vi "main(Test DQMH modules).vi"() -> ()   [LabVIEW 2018, in "Application.lvlib"] (continued)
        n2137 = Build Array(w5001, w5000, w4999) -> (w5007:T9[])
        n2138 = for {
          tunnel: [w5039] -> w5013 mode=indexing
          shift-right: [w5040] -> w5015
          shift-left: w5008 -> [w5038]
          tunnel: w5007 -> [w5037] mode=indexing
          n2139 = Unbundle By Name(w5037) -> ("command"=w5036:string, "data"=w5035:variant)
          n2140 = call "App enquece.vi"("Priority Enquece"=TRUE, "command data"=w5035, "command"=w5036, "queue in"=w5038) -> ("error out"=w5039:errorcluster, "Queue out"=w5040:refnum<queue>)  [unwired: 6 in]
        }
        n2141 = call "FGV DRV stand.vi"() -> ("Sub-Test.DCV"=w4996:bool)  [unwired: 10 in, 1 out]
        n2142 = case shown="True" w4996 {
          tunnel: [w5026 w5034] -> w5016
          frame False {
            n2143 = Build Array("WaitFor", "MEAS.requestAC") -> (w5026:string[])
          }
          frame True {
            n2144 = Build Array("Test DRV 1", "Test DRV 2", "Test DRV 3", "WaitForC", "MEAS.requestAC") -> (w5034:string[])
          }
        }
        n2145 = Merge Errors(w5013) -> (w5006:errorcluster)
        n2146 = Reverse 1D Array(array=w5016) -> (reversed array=w4995:string[])
        n2147 = for {
          tunnel: w4995 -> [w5046] mode=indexing
          tunnel: [w5045] -> w5012 mode=indexing
          shift-right: [w5044] -> w5014
          shift-left: w5015 -> [w5047]
          tunnel: w5006 -> [w5043]
          n2148 = call "App enquece.vi"("Priority Enquece"=TRUE, "error in (no error)"=w5043, "command"=w5046, "queue in"=w5047) -> ("error out"=w5045:errorcluster, "Queue out"=w5044:refnum<queue>)  [unwired: 6 in]
        }
        n2149 = Merge Errors(w5012) -> (w5011:errorcluster)
        n2150 = Initialize Array(FALSE ("element"), 6 ("dimension size")) -> (w4977:bool[])
        n2151 = Initialize Array(TRUE, 3 ("dimension size")) -> (w4976:bool[])
        n2152 = Replace Array Subset(array=w4977, new element=w4976) -> (w4975:bool[])  [unwired: 1 in]
        n2153 = To Variant(anything=T3."mux10_1_channel1" ("mux10_1(x6)_encode")) -> (Variant=w4992:variant)
        n2154 = To Variant(anything=T4."demux1_10_channel1" ("demux1_10(x6)_encode")) -> (Variant=w4988:variant)
        n2155 = To Variant(anything=w4975) -> (Variant=w4984:variant)
        n2156 = Bundle By Name(cluster=w4981, "command"="MEAS.mux10-1", "data"=w4992) -> (w4987:T9)
        n2157 = Bundle By Name(cluster=w4981, "command"="MEAS.demux1-10", "data"=w4988) -> (w4986:T9)
        n2158 = Bundle By Name(cluster=w4981, "command"="MEAS.eMIC", "data"=w4984) -> (w4983:T9)
        n2159 = Build Array(w4987, w4986, w4983) -> (w5010:T9[])
        n2160 = Reverse 1D Array(array=w5010) -> (reversed array=w5009:T9[])
        n2161 = for {
          tunnel: w5009 -> [w5057] mode=indexing
          tunnel: [w5054] -> w5017 mode=indexing
          tunnel: w5011 -> [w5053]
          tunnel: w5014 -> [w5058]
          n2162 = Unbundle By Name(w5057) -> ("command"=w5056:string, "data"=w5055:variant)
          n2163 = call "App enquece.vi"("Priority Enquece"=TRUE, "error in (no error)"=w5053, "command data"=w5055, "command"=w5056, "queue in"=w5058) -> ("error out"=w5054:errorcluster)  [unwired: 5 in, 1 out]
        }
        n2164 = Merge Errors(w5020, w5017) -> (w5021:errorcluster)
      }
      frame "Test Channel 2C" {
        w5065 = T9 {"command"="", "data"=variant} ("element")
        w5086 = T9 {"command"="", "data"=variant} ("element")
        w5107 = 2  # DUT channel (1-10)
        n2165 = disable-structure shown="LOGGING==TRUE" {
          disable-tunnel: w5102 -> [w5133 _]
          frame condition #0 (active) {
            n2166 = Empty String/Path?(string/path=w5133) -> (empty?=w5135:bool)
            n2167 = Select(t="Quece timeout", s=w5135, f=w5133) -> (s? t:f=w5132:string)
            n2168 = call "string log (SubVI).vi"("state Name"=w5132) -> ()  [unwired: 9 in, 2 out]
          }
          frame condition #1 {
          }
        }
        n2169 = Bundle By Name(cluster=w5086, "command"="Apps.UI Update", "data"="C") -> (w5085:T9)
        n2170 = Bundle By Name(cluster=w5086, "command"="MEAS.AllRelaysOFF2") -> (w5084:T9)
        n2171 = Bundle By Name(cluster=w5086, "command"="Apps.WaitForEvent") -> (w5083:T9)
        n2172 = Build Array(w5085, w5084, w5083) -> (w5091:T9[])
        n2173 = for {
          tunnel: [w5123] -> w5097 mode=indexing
          shift-right: [w5124] -> w5099
          shift-left: w5092 -> [w5122]
          tunnel: w5091 -> [w5121] mode=indexing
          n2174 = Unbundle By Name(w5121) -> ("command"=w5120:string, "data"=w5119:variant)
          n2175 = call "App enquece.vi"("Priority Enquece"=TRUE, "command data"=w5119, "command"=w5120, "queue in"=w5122) -> ("error out"=w5123:errorcluster, "Queue out"=w5124:refnum<queue>)  [unwired: 6 in]
        }
        n2176 = call "FGV DRV stand.vi"() -> ("Sub-Test.DCV"=w5080:bool)  [unwired: 10 in, 1 out]
        n2177 = case shown="True" w5080 {
          tunnel: [w5110 w5118] -> w5100
          frame False {
            n2178 = Build Array("WaitFor", "MEAS.requestAC") -> (w5110:string[])
          }
          frame True {
            n2179 = Build Array("Test DRV 7", "Test DRV 8", "Test DRV 9", "WaitForC", "MEAS.requestAC") -> (w5118:string[])
          }
        }
        n2180 = Merge Errors(w5097) -> (w5090:errorcluster)
        n2181 = Reverse 1D Array(array=w5100) -> (reversed array=w5079:string[])
        n2182 = for {
          tunnel: w5079 -> [w5130] mode=indexing
          tunnel: [w5129] -> w5096 mode=indexing
          shift-right: [w5128] -> w5098
          shift-left: w5099 -> [w5131]
          tunnel: w5090 -> [w5127]
          n2183 = call "App enquece.vi"("Priority Enquece"=TRUE, "error in (no error)"=w5127, "command"=w5130, "queue in"=w5131) -> ("error out"=w5129:errorcluster, "Queue out"=w5128:refnum<queue>)  [unwired: 6 in]
        }
        n2184 = Initialize Array(FALSE ("element"), 6 ("dimension size")) -> (w5061:bool[])
        n2185 = Initialize Array(TRUE, 3 ("dimension size")) -> (w5060:bool[])
        n2186 = Merge Errors(w5096) -> (w5095:errorcluster)
        n2187 = Replace Array Subset(array=w5061, new element=w5060) -> (w5059:bool[])  [unwired: 1 in]
        n2188 = To Variant(anything=T3."mux10_1_channel2" ("mux10_1(x6)_encode")) -> (Variant=w5076:variant)
        n2189 = To Variant(anything=T4."demux1_10_channel2" ("demux1_10(x6)_encode")) -> (Variant=w5072:variant)
        n2190 = To Variant(anything=w5059) -> (Variant=w5068:variant)
        n2191 = Bundle By Name(cluster=w5065, "command"="MEAS.mux10-1", "data"=w5076) -> (w5071:T9)
        n2192 = Bundle By Name(cluster=w5065, "command"="MEAS.demux1-10", "data"=w5072) -> (w5070:T9)
        n2193 = Bundle By Name(cluster=w5065, "command"="MEAS.eMIC", "data"=w5068) -> (w5067:T9)
        n2194 = Build Array(w5071, w5070, w5067) -> (w5094:T9[])
        n2195 = Reverse 1D Array(array=w5094) -> (reversed array=w5093:T9[])
        n2196 = for {
          tunnel: w5093 -> [w5141] mode=indexing
          tunnel: [w5138] -> w5101 mode=indexing
          tunnel: w5095 -> [w5137]
          tunnel: w5098 -> [w5142]
          n2197 = Unbundle By Name(w5141) -> ("command"=w5140:string, "data"=w5139:variant)
          n2198 = call "App enquece.vi"("Priority Enquece"=TRUE, "error in (no error)"=w5137, "command data"=w5139, "command"=w5140, "queue in"=w5142) -> ("error out"=w5138:errorcluster)  [unwired: 5 in, 1 out]
        }
        n2199 = Merge Errors(w5104, w5101) -> (w5105:errorcluster)
      }
      frame "Test Channel 3C" {
        w5149 = T9 {"command"="", "data"=variant} ("element")
        w5170 = T9 {"command"="", "data"=variant} ("element")
        w5191 = 3  # DUT channel (1-10)
        n2200 = disable-structure shown="LOGGING==TRUE" {
          disable-tunnel: w5186 -> [w5217 _]
          frame condition #0 (active) {
            n2201 = Empty String/Path?(string/path=w5217) -> (empty?=w5219:bool)
            n2202 = Select(t="Quece timeout", s=w5219, f=w5217) -> (s? t:f=w5216:string)
            n2203 = call "string log (SubVI).vi"("state Name"=w5216) -> ()  [unwired: 9 in, 2 out]
          }
          frame condition #1 {
          }
        }
        n2204 = Bundle By Name(cluster=w5170, "command"="Apps.UI Update", "data"="C") -> (w5169:T9)
        n2205 = Bundle By Name(cluster=w5170, "command"="MEAS.AllRelaysOFF2") -> (w5168:T9)
        n2206 = Bundle By Name(cluster=w5170, "command"="Apps.WaitForEvent") -> (w5167:T9)
        n2207 = Build Array(w5169, w5168, w5167) -> (w5175:T9[])
        n2208 = for {
          tunnel: [w5207] -> w5181 mode=indexing
          shift-right: [w5208] -> w5183
          shift-left: w5176 -> [w5206]
          tunnel: w5175 -> [w5205] mode=indexing
          n2209 = Unbundle By Name(w5205) -> ("command"=w5204:string, "data"=w5203:variant)
          n2210 = call "App enquece.vi"("Priority Enquece"=TRUE, "command data"=w5203, "command"=w5204, "queue in"=w5206) -> ("error out"=w5207:errorcluster, "Queue out"=w5208:refnum<queue>)  [unwired: 6 in]
        }
        n2211 = call "FGV DRV stand.vi"() -> ("Sub-Test.DCV"=w5164:bool)  [unwired: 10 in, 1 out]
        n2212 = case shown="False" w5164 {
          tunnel: [w5194 w5202] -> w5184
          frame False {
            n2213 = Build Array("WaitFor", "MEAS.requestAC") -> (w5194:string[])
          }
          frame True {
            n2214 = Build Array("Test DRV 13", "Test DRV 14", "Test DRV 15", "WaitForC", "MEAS.requestAC") -> (w5202:string[])
          }
        }
        n2215 = Merge Errors(w5181) -> (w5174:errorcluster)
        n2216 = Reverse 1D Array(array=w5184) -> (reversed array=w5163:string[])
        n2217 = for {
          tunnel: w5163 -> [w5214] mode=indexing
          tunnel: [w5213] -> w5180 mode=indexing
          shift-right: [w5212] -> w5182
          shift-left: w5183 -> [w5215]
          tunnel: w5174 -> [w5211]
          n2218 = call "App enquece.vi"("Priority Enquece"=TRUE, "error in (no error)"=w5211, "command"=w5214, "queue in"=w5215) -> ("error out"=w5213:errorcluster, "Queue out"=w5212:refnum<queue>)  [unwired: 6 in]
        }
        n2219 = Merge Errors(w5180) -> (w5179:errorcluster)
        n2220 = Initialize Array(FALSE ("element"), 6 ("dimension size")) -> (w5145:bool[])
        n2221 = Initialize Array(TRUE, 3 ("dimension size")) -> (w5144:bool[])
        n2222 = Replace Array Subset(array=w5145, new element=w5144) -> (w5143:bool[])  [unwired: 1 in]
        n2223 = To Variant(anything=T3."mux10_1_channel3" ("mux10_1(x6)_encode")) -> (Variant=w5160:variant)
        n2224 = To Variant(anything=T4."demux1_10_channel3" ("demux1_10(x6)_encode")) -> (Variant=w5156:variant)
        n2225 = To Variant(anything=w5143) -> (Variant=w5152:variant)
        n2226 = Bundle By Name(cluster=w5149, "command"="MEAS.mux10-1", "data"=w5160) -> (w5155:T9)
        n2227 = Bundle By Name(cluster=w5149, "command"="MEAS.demux1-10", "data"=w5156) -> (w5154:T9)
        n2228 = Bundle By Name(cluster=w5149, "command"="MEAS.eMIC", "data"=w5152) -> (w5151:T9)
        n2229 = Build Array(w5155, w5154, w5151) -> (w5178:T9[])
        n2230 = Reverse 1D Array(array=w5178) -> (reversed array=w5177:T9[])
        n2231 = for {
          tunnel: w5177 -> [w5225] mode=indexing
          tunnel: [w5222] -> w5185 mode=indexing
          tunnel: w5179 -> [w5221]
          tunnel: w5182 -> [w5226]
          n2232 = Unbundle By Name(w5225) -> ("command"=w5224:string, "data"=w5223:variant)
          n2233 = call "App enquece.vi"("Priority Enquece"=TRUE, "error in (no error)"=w5221, "command data"=w5223, "command"=w5224, "queue in"=w5226) -> ("error out"=w5222:errorcluster)  [unwired: 5 in, 1 out]
        }
        n2234 = Merge Errors(w5188, w5185) -> (w5189:errorcluster)
      }
      frame "Test Channel 4C" {
        w5233 = T9 {"command"="", "data"=variant} ("element")
        w5254 = T9 {"command"="", "data"=variant} ("element")
        w5275 = 4  # DUT channel (1-10)
        n2235 = disable-structure shown="LOGGING==TRUE" {
          disable-tunnel: w5270 -> [w5301 _]
          frame condition #0 (active) {
            n2236 = Empty String/Path?(string/path=w5301) -> (empty?=w5303:bool)
            n2237 = Select(t="Quece timeout", s=w5303, f=w5301) -> (s? t:f=w5300:string)
            n2238 = call "string log (SubVI).vi"("state Name"=w5300) -> ()  [unwired: 9 in, 2 out]
          }
          frame condition #1 {
          }
        }
        n2239 = Bundle By Name(cluster=w5254, "command"="Apps.UI Update", "data"="C") -> (w5253:T9)
        n2240 = Bundle By Name(cluster=w5254, "command"="MEAS.AllRelaysOFF2") -> (w5252:T9)
        n2241 = Bundle By Name(cluster=w5254, "command"="Apps.WaitForEvent") -> (w5251:T9)
        n2242 = Build Array(w5253, w5252, w5251) -> (w5259:T9[])
        n2243 = for {
          tunnel: [w5291] -> w5265 mode=indexing
          shift-right: [w5292] -> w5267
          shift-left: w5260 -> [w5290]
          tunnel: w5259 -> [w5289] mode=indexing
          n2244 = Unbundle By Name(w5289) -> ("command"=w5288:string, "data"=w5287:variant)
          n2245 = call "App enquece.vi"("Priority Enquece"=TRUE, "command data"=w5287, "command"=w5288, "queue in"=w5290) -> ("error out"=w5291:errorcluster, "Queue out"=w5292:refnum<queue>)  [unwired: 6 in]
        }
        n2246 = call "FGV DRV stand.vi"() -> ("Sub-Test.DCV"=w5248:bool)  [unwired: 10 in, 1 out]
        n2247 = case shown="True" w5248 {
          tunnel: [w5278 w5286] -> w5268
          frame False {
            n2248 = Build Array("WaitFor", "MEAS.requestAC") -> (w5278:string[])
          }
          frame True {
            n2249 = Build Array("Test DRV 19", "Test DRV 20", "Test DRV 21", "WaitForC", "MEAS.requestAC") -> (w5286:string[])
          }
        }
        n2250 = Merge Errors(w5265) -> (w5258:errorcluster)
        n2251 = Reverse 1D Array(array=w5268) -> (reversed array=w5247:string[])
        n2252 = for {
          tunnel: w5247 -> [w5298] mode=indexing
          tunnel: [w5297] -> w5264 mode=indexing
          shift-right: [w5296] -> w5266
          shift-left: w5267 -> [w5299]
          tunnel: w5258 -> [w5295]
          n2253 = call "App enquece.vi"("Priority Enquece"=TRUE, "error in (no error)"=w5295, "command"=w5298, "queue in"=w5299) -> ("error out"=w5297:errorcluster, "Queue out"=w5296:refnum<queue>)  [unwired: 6 in]
        }
        n2254 = Initialize Array(FALSE ("element"), 6 ("dimension size")) -> (w5229:bool[])
        n2255 = Initialize Array(TRUE, 3 ("dimension size")) -> (w5228:bool[])
        n2256 = Merge Errors(w5264) -> (w5263:errorcluster)
        n2257 = Replace Array Subset(array=w5229, new element=w5228) -> (w5227:bool[])  [unwired: 1 in]
        n2258 = To Variant(anything=T3."mux10_1_channel4" ("mux10_1(x6)_encode")) -> (Variant=w5244:variant)
        n2259 = To Variant(anything=T4."demux1_10_channel4" ("demux1_10(x6)_encode")) -> (Variant=w5240:variant)
        n2260 = To Variant(anything=w5227) -> (Variant=w5236:variant)
        n2261 = Bundle By Name(cluster=w5233, "command"="MEAS.mux10-1", "data"=w5244) -> (w5239:T9)
        n2262 = Bundle By Name(cluster=w5233, "command"="MEAS.demux1-10", "data"=w5240) -> (w5238:T9)
        n2263 = Bundle By Name(cluster=w5233, "command"="MEAS.eMIC", "data"=w5236) -> (w5235:T9)
        n2264 = Build Array(w5239, w5238, w5235) -> (w5262:T9[])
        n2265 = Reverse 1D Array(array=w5262) -> (reversed array=w5261:T9[])
        n2266 = for {
          tunnel: w5261 -> [w5309] mode=indexing
          tunnel: [w5306] -> w5269 mode=indexing
          tunnel: w5263 -> [w5305]
          tunnel: w5266 -> [w5310]
          n2267 = Unbundle By Name(w5309) -> ("command"=w5308:string, "data"=w5307:variant)
          n2268 = call "App enquece.vi"("Priority Enquece"=TRUE, "error in (no error)"=w5305, "command data"=w5307, "command"=w5308, "queue in"=w5310) -> ("error out"=w5306:errorcluster)  [unwired: 5 in, 1 out]
        }
        n2269 = Merge Errors(w5272, w5269) -> (w5273:errorcluster)
      }
      frame "Test Channel 5C" {
        w5317 = T9 {"command"="", "data"=variant} ("element")
        w5338 = T9 {"command"="", "data"=variant} ("element")
        w5359 = 5  # DUT channel (1-10)
        n2270 = disable-structure shown="LOGGING==TRUE" {
          disable-tunnel: w5354 -> [w5385 _]
          frame condition #0 (active) {
            n2271 = Empty String/Path?(string/path=w5385) -> (empty?=w5387:bool)
            n2272 = Select(t="Quece timeout", s=w5387, f=w5385) -> (s? t:f=w5384:string)
            n2273 = call "string log (SubVI).vi"("state Name"=w5384) -> ()  [unwired: 9 in, 2 out]
          }
          frame condition #1 {
          }
        }
        n2274 = Bundle By Name(cluster=w5338, "command"="Apps.UI Update", "data"="C") -> (w5337:T9)
        n2275 = Bundle By Name(cluster=w5338, "command"="MEAS.AllRelaysOFF2") -> (w5336:T9)
        n2276 = Bundle By Name(cluster=w5338, "command"="Apps.WaitForEvent") -> (w5335:T9)
        n2277 = Build Array(w5337, w5336, w5335) -> (w5343:T9[])
        n2278 = for {
          tunnel: [w5375] -> w5349 mode=indexing
          shift-right: [w5376] -> w5351
          shift-left: w5344 -> [w5374]
          tunnel: w5343 -> [w5373] mode=indexing
          n2279 = Unbundle By Name(w5373) -> ("command"=w5372:string, "data"=w5371:variant)
          n2280 = call "App enquece.vi"("Priority Enquece"=TRUE, "command data"=w5371, "command"=w5372, "queue in"=w5374) -> ("error out"=w5375:errorcluster, "Queue out"=w5376:refnum<queue>)  [unwired: 6 in]
        }
        n2281 = call "FGV DRV stand.vi"() -> ("Sub-Test.DCV"=w5332:bool)  [unwired: 10 in, 1 out]
        n2282 = case shown="False" w5332 {
          tunnel: [w5362 w5370] -> w5352
          frame False {
            n2283 = Build Array("WaitFor", "MEAS.requestAC") -> (w5362:string[])
          }
          frame True {
            n2284 = Build Array("Test DRV 25", "Test DRV 26", "Test DRV 27", "WaitForC", "MEAS.requestAC") -> (w5370:string[])
          }
        }
        n2285 = Merge Errors(w5349) -> (w5342:errorcluster)
        n2286 = Reverse 1D Array(array=w5352) -> (reversed array=w5331:string[])
        n2287 = for {
          tunnel: w5331 -> [w5382] mode=indexing
          tunnel: [w5381] -> w5348 mode=indexing
          shift-right: [w5380] -> w5350
          shift-left: w5351 -> [w5383]
          tunnel: w5342 -> [w5379]
          n2288 = call "App enquece.vi"("Priority Enquece"=TRUE, "error in (no error)"=w5379, "command"=w5382, "queue in"=w5383) -> ("error out"=w5381:errorcluster, "Queue out"=w5380:refnum<queue>)  [unwired: 6 in]
        }
        n2289 = Merge Errors(w5348) -> (w5347:errorcluster)
        n2290 = Initialize Array(FALSE ("element"), 6 ("dimension size")) -> (w5313:bool[])
        n2291 = Initialize Array(TRUE, 3 ("dimension size")) -> (w5312:bool[])
        n2292 = Replace Array Subset(array=w5313, new element=w5312) -> (w5311:bool[])  [unwired: 1 in]
        n2293 = To Variant(anything=T3."mux10_1_channel5" ("mux10_1(x6)_encode")) -> (Variant=w5328:variant)
        n2294 = To Variant(anything=T4."demux1_10_channel5" ("demux1_10(x6)_encode")) -> (Variant=w5324:variant)
        n2295 = To Variant(anything=w5311) -> (Variant=w5320:variant)
        n2296 = Bundle By Name(cluster=w5317, "command"="MEAS.mux10-1", "data"=w5328) -> (w5323:T9)
        n2297 = Bundle By Name(cluster=w5317, "command"="MEAS.demux1-10", "data"=w5324) -> (w5322:T9)
        n2298 = Bundle By Name(cluster=w5317, "command"="MEAS.eMIC", "data"=w5320) -> (w5319:T9)
        n2299 = Build Array(w5323, w5322, w5319) -> (w5346:T9[])
        n2300 = Reverse 1D Array(array=w5346) -> (reversed array=w5345:T9[])
        n2301 = for {
          tunnel: w5345 -> [w5393] mode=indexing
          tunnel: [w5390] -> w5353 mode=indexing
          tunnel: w5347 -> [w5389]
          tunnel: w5350 -> [w5394]
          n2302 = Unbundle By Name(w5393) -> ("command"=w5392:string, "data"=w5391:variant)
          n2303 = call "App enquece.vi"("Priority Enquece"=TRUE, "error in (no error)"=w5389, "command data"=w5391, "command"=w5392, "queue in"=w5394) -> ("error out"=w5390:errorcluster)  [unwired: 5 in, 1 out]
        }
        n2304 = Merge Errors(w5356, w5353) -> (w5357:errorcluster)
      }
      frame "Test Channel 6C" {
        w5401 = T9 {"command"="", "data"=variant} ("element")
        w5422 = T9 {"command"="", "data"=variant} ("element")
        w5443 = 6  # DUT channel (1-10)
        n2305 = disable-structure shown="LOGGING==TRUE" {
          disable-tunnel: w5438 -> [w5469 _]
          frame condition #0 (active) {
            n2306 = Empty String/Path?(string/path=w5469) -> (empty?=w5471:bool)
            n2307 = Select(t="Quece timeout", s=w5471, f=w5469) -> (s? t:f=w5468:string)
            n2308 = call "string log (SubVI).vi"("state Name"=w5468) -> ()  [unwired: 9 in, 2 out]
          }
          frame condition #1 {
          }
        }
        n2309 = Bundle By Name(cluster=w5422, "command"="Apps.UI Update", "data"="C") -> (w5421:T9)
        n2310 = Bundle By Name(cluster=w5422, "command"="MEAS.AllRelaysOFF2") -> (w5420:T9)
        n2311 = Bundle By Name(cluster=w5422, "command"="Apps.WaitForEvent") -> (w5419:T9)
        n2312 = Build Array(w5421, w5420, w5419) -> (w5427:T9[])
        n2313 = for {
          tunnel: [w5459] -> w5433 mode=indexing
          shift-right: [w5460] -> w5435
          shift-left: w5428 -> [w5458]
          tunnel: w5427 -> [w5457] mode=indexing
          n2314 = Unbundle By Name(w5457) -> ("command"=w5456:string, "data"=w5455:variant)
          n2315 = call "App enquece.vi"("Priority Enquece"=TRUE, "command data"=w5455, "command"=w5456, "queue in"=w5458) -> ("error out"=w5459:errorcluster, "Queue out"=w5460:refnum<queue>)  [unwired: 6 in]
        }
        n2316 = call "FGV DRV stand.vi"() -> ("Sub-Test.DCV"=w5416:bool)  [unwired: 10 in, 1 out]
        n2317 = case shown="False" w5416 {
          tunnel: [w5446 w5454] -> w5436
          frame False {
            n2318 = Build Array("WaitFor", "MEAS.requestAC") -> (w5446:string[])
          }
          frame True {
            n2319 = Build Array("Test DRV 31", "Test DRV 32", "Test DRV 33", "WaitForC", "MEAS.requestAC") -> (w5454:string[])
          }
        }
        n2320 = Merge Errors(w5433) -> (w5426:errorcluster)
        n2321 = Reverse 1D Array(array=w5436) -> (reversed array=w5415:string[])
        n2322 = for {
          tunnel: w5415 -> [w5466] mode=indexing
          tunnel: [w5465] -> w5432 mode=indexing
          shift-right: [w5464] -> w5434
          shift-left: w5435 -> [w5467]
          tunnel: w5426 -> [w5463]
          n2323 = call "App enquece.vi"("Priority Enquece"=TRUE, "error in (no error)"=w5463, "command"=w5466, "queue in"=w5467) -> ("error out"=w5465:errorcluster, "Queue out"=w5464:refnum<queue>)  [unwired: 6 in]
        }
        n2324 = Initialize Array(FALSE ("element"), 6 ("dimension size")) -> (w5397:bool[])
        n2325 = Initialize Array(TRUE, 3 ("dimension size")) -> (w5396:bool[])
        n2326 = Merge Errors(w5432) -> (w5431:errorcluster)
        n2327 = Replace Array Subset(array=w5397, new element=w5396) -> (w5395:bool[])  [unwired: 1 in]
        n2328 = To Variant(anything=T3."mux10_1_channel6" ("mux10_1(x6)_encode")) -> (Variant=w5412:variant)
        n2329 = To Variant(anything=T4."demux1_10_channel6" ("demux1_10(x6)_encode")) -> (Variant=w5408:variant)
        n2330 = To Variant(anything=w5395) -> (Variant=w5404:variant)
        n2331 = Bundle By Name(cluster=w5401, "command"="MEAS.mux10-1", "data"=w5412) -> (w5407:T9)
        n2332 = Bundle By Name(cluster=w5401, "command"="MEAS.demux1-10", "data"=w5408) -> (w5406:T9)
        n2333 = Bundle By Name(cluster=w5401, "command"="MEAS.eMIC", "data"=w5404) -> (w5403:T9)
        n2334 = Build Array(w5407, w5406, w5403) -> (w5430:T9[])
        n2335 = Reverse 1D Array(array=w5430) -> (reversed array=w5429:T9[])
        n2336 = for {
          tunnel: w5429 -> [w5477] mode=indexing
          tunnel: [w5474] -> w5437 mode=indexing
          tunnel: w5431 -> [w5473]
          tunnel: w5434 -> [w5478]
          n2337 = Unbundle By Name(w5477) -> ("command"=w5476:string, "data"=w5475:variant)
          n2338 = call "App enquece.vi"("Priority Enquece"=TRUE, "error in (no error)"=w5473, "command data"=w5475, "command"=w5476, "queue in"=w5478) -> ("error out"=w5474:errorcluster)  [unwired: 5 in, 1 out]
        }
        n2339 = Merge Errors(w5440, w5437) -> (w5441:errorcluster)
      }
      frame "Test Channel 7C" {
        w5485 = T9 {"command"="", "data"=variant} ("element")
        w5506 = T9 {"command"="", "data"=variant} ("element")
        w5527 = 7  # DUT channel (1-10)
        n2340 = disable-structure shown="LOGGING==TRUE" {
          disable-tunnel: w5522 -> [w5553 _]
          frame condition #0 (active) {
            n2341 = Empty String/Path?(string/path=w5553) -> (empty?=w5555:bool)
            n2342 = Select(t="Quece timeout", s=w5555, f=w5553) -> (s? t:f=w5552:string)
            n2343 = call "string log (SubVI).vi"("state Name"=w5552) -> ()  [unwired: 9 in, 2 out]
          }
          frame condition #1 {
          }
        }
        n2344 = Bundle By Name(cluster=w5506, "command"="Apps.UI Update", "data"="C") -> (w5505:T9)
        n2345 = Bundle By Name(cluster=w5506, "command"="MEAS.AllRelaysOFF2") -> (w5504:T9)
        n2346 = Bundle By Name(cluster=w5506, "command"="Apps.WaitForEvent") -> (w5503:T9)
        n2347 = Build Array(w5505, w5504, w5503) -> (w5511:T9[])
        n2348 = for {
          tunnel: [w5543] -> w5517 mode=indexing
          shift-right: [w5544] -> w5519
          shift-left: w5512 -> [w5542]
          tunnel: w5511 -> [w5541] mode=indexing
          n2349 = Unbundle By Name(w5541) -> ("command"=w5540:string, "data"=w5539:variant)
          n2350 = call "App enquece.vi"("Priority Enquece"=TRUE, "command data"=w5539, "command"=w5540, "queue in"=w5542) -> ("error out"=w5543:errorcluster, "Queue out"=w5544:refnum<queue>)  [unwired: 6 in]
        }
        n2351 = call "FGV DRV stand.vi"() -> ("Sub-Test.DCV"=w5500:bool)  [unwired: 10 in, 1 out]
        n2352 = case shown="False" w5500 {
          tunnel: [w5530 w5538] -> w5520
          frame False {
            n2353 = Build Array("WaitFor", "MEAS.requestAC") -> (w5530:string[])
          }
          frame True {
            n2354 = Build Array("Test DRV 37", "Test DRV 38", "Test DRV 39", "WaitForC", "MEAS.requestAC") -> (w5538:string[])
          }
        }
        n2355 = Merge Errors(w5517) -> (w5510:errorcluster)
        n2356 = Reverse 1D Array(array=w5520) -> (reversed array=w5499:string[])
        n2357 = for {
          tunnel: w5499 -> [w5550] mode=indexing
          tunnel: [w5549] -> w5516 mode=indexing
          shift-right: [w5548] -> w5518
          shift-left: w5519 -> [w5551]
          tunnel: w5510 -> [w5547]
          n2358 = call "App enquece.vi"("Priority Enquece"=TRUE, "error in (no error)"=w5547, "command"=w5550, "queue in"=w5551) -> ("error out"=w5549:errorcluster, "Queue out"=w5548:refnum<queue>)  [unwired: 6 in]
        }
        n2359 = Initialize Array(FALSE ("element"), 6 ("dimension size")) -> (w5481:bool[])
        n2360 = Initialize Array(TRUE, 3 ("dimension size")) -> (w5480:bool[])
        n2361 = Merge Errors(w5516) -> (w5515:errorcluster)
        n2362 = Replace Array Subset(array=w5481, new element=w5480) -> (w5479:bool[])  [unwired: 1 in]
        n2363 = To Variant(anything=T3."mux10_1_channel7" ("mux10_1(x6)_encode")) -> (Variant=w5496:variant)
        n2364 = To Variant(anything=T4."demux1_10_channel7" ("demux1_10(x6)_encode")) -> (Variant=w5492:variant)
        n2365 = To Variant(anything=w5479) -> (Variant=w5488:variant)
        n2366 = Bundle By Name(cluster=w5485, "command"="MEAS.mux10-1", "data"=w5496) -> (w5491:T9)
        n2367 = Bundle By Name(cluster=w5485, "command"="MEAS.demux1-10", "data"=w5492) -> (w5490:T9)
        n2368 = Bundle By Name(cluster=w5485, "command"="MEAS.eMIC", "data"=w5488) -> (w5487:T9)
        n2369 = Build Array(w5491, w5490, w5487) -> (w5514:T9[])
        n2370 = Reverse 1D Array(array=w5514) -> (reversed array=w5513:T9[])
        n2371 = for {
          tunnel: w5513 -> [w5561] mode=indexing
          tunnel: [w5558] -> w5521 mode=indexing
          tunnel: w5515 -> [w5557]
          tunnel: w5518 -> [w5562]
          n2372 = Unbundle By Name(w5561) -> ("command"=w5560:string, "data"=w5559:variant)
          n2373 = call "App enquece.vi"("Priority Enquece"=TRUE, "error in (no error)"=w5557, "command data"=w5559, "command"=w5560, "queue in"=w5562) -> ("error out"=w5558:errorcluster)  [unwired: 5 in, 1 out]
        }
        n2374 = Merge Errors(w5524, w5521) -> (w5525:errorcluster)
      }
      frame "Test Channel 8C" {
        w5569 = T9 {"command"="", "data"=variant} ("element")
        w5590 = T9 {"command"="", "data"=variant} ("element")
        w5611 = 8  # DUT channel (1-10)
        n2375 = disable-structure shown="LOGGING==TRUE" {
          disable-tunnel: w5606 -> [w5637 _]
          frame condition #0 (active) {
            n2376 = Empty String/Path?(string/path=w5637) -> (empty?=w5639:bool)
            n2377 = Select(t="Quece timeout", s=w5639, f=w5637) -> (s? t:f=w5636:string)
            n2378 = call "string log (SubVI).vi"("state Name"=w5636) -> ()  [unwired: 9 in, 2 out]
          }
          frame condition #1 {
          }
        }
        n2379 = Bundle By Name(cluster=w5590, "command"="Apps.UI Update", "data"="C") -> (w5589:T9)
        n2380 = Bundle By Name(cluster=w5590, "command"="MEAS.AllRelaysOFF2") -> (w5588:T9)
        n2381 = Bundle By Name(cluster=w5590, "command"="Apps.WaitForEvent") -> (w5587:T9)
        n2382 = Build Array(w5589, w5588, w5587) -> (w5595:T9[])
        n2383 = for {
          tunnel: [w5627] -> w5601 mode=indexing
          shift-right: [w5628] -> w5603
          shift-left: w5596 -> [w5626]
          tunnel: w5595 -> [w5625] mode=indexing
          n2384 = Unbundle By Name(w5625) -> ("command"=w5624:string, "data"=w5623:variant)
          n2385 = call "App enquece.vi"("Priority Enquece"=TRUE, "command data"=w5623, "command"=w5624, "queue in"=w5626) -> ("error out"=w5627:errorcluster, "Queue out"=w5628:refnum<queue>)  [unwired: 6 in]
        }
        n2386 = call "FGV DRV stand.vi"() -> ("Sub-Test.DCV"=w5584:bool)  [unwired: 10 in, 1 out]
        n2387 = case shown="True" w5584 {
          tunnel: [w5614 w5622] -> w5604
          frame False {
            n2388 = Build Array("WaitFor", "MEAS.requestAC") -> (w5614:string[])
          }
          frame True {
            n2389 = Build Array("Test DRV 43", "Test DRV 44", "Test DRV 45", "WaitForC", "MEAS.requestAC") -> (w5622:string[])
          }
        }
        n2390 = Merge Errors(w5601) -> (w5594:errorcluster)
        n2391 = Reverse 1D Array(array=w5604) -> (reversed array=w5583:string[])
        n2392 = for {
          tunnel: w5583 -> [w5634] mode=indexing
          tunnel: [w5633] -> w5600 mode=indexing
          shift-right: [w5632] -> w5602
          shift-left: w5603 -> [w5635]
          tunnel: w5594 -> [w5631]
          n2393 = call "App enquece.vi"("Priority Enquece"=TRUE, "error in (no error)"=w5631, "command"=w5634, "queue in"=w5635) -> ("error out"=w5633:errorcluster, "Queue out"=w5632:refnum<queue>)  [unwired: 6 in]
        }
        n2394 = Initialize Array(FALSE ("element"), 6 ("dimension size")) -> (w5565:bool[])
        n2395 = Initialize Array(TRUE, 3 ("dimension size")) -> (w5564:bool[])
        n2396 = Merge Errors(w5600) -> (w5599:errorcluster)
        n2397 = Replace Array Subset(array=w5565, new element=w5564) -> (w5563:bool[])  [unwired: 1 in]
        n2398 = To Variant(anything=T3."mux10_1_channel8" ("mux10_1(x6)_encode")) -> (Variant=w5580:variant)
        n2399 = To Variant(anything=T4."demux1_10_channel8" ("demux1_10(x6)_encode")) -> (Variant=w5576:variant)
        n2400 = To Variant(anything=w5563) -> (Variant=w5572:variant)
        n2401 = Bundle By Name(cluster=w5569, "command"="MEAS.mux10-1", "data"=w5580) -> (w5575:T9)
        n2402 = Bundle By Name(cluster=w5569, "command"="MEAS.demux1-10", "data"=w5576) -> (w5574:T9)
        n2403 = Bundle By Name(cluster=w5569, "command"="MEAS.eMIC", "data"=w5572) -> (w5571:T9)
        n2404 = Build Array(w5575, w5574, w5571) -> (w5598:T9[])
        n2405 = Reverse 1D Array(array=w5598) -> (reversed array=w5597:T9[])
        n2406 = for {
          tunnel: w5597 -> [w5645] mode=indexing
          tunnel: [w5642] -> w5605 mode=indexing
          tunnel: w5599 -> [w5641]
          tunnel: w5602 -> [w5646]
          n2407 = Unbundle By Name(w5645) -> ("command"=w5644:string, "data"=w5643:variant)
          n2408 = call "App enquece.vi"("Priority Enquece"=TRUE, "error in (no error)"=w5641, "command data"=w5643, "command"=w5644, "queue in"=w5646) -> ("error out"=w5642:errorcluster)  [unwired: 5 in, 1 out]
        }
        n2409 = Merge Errors(w5608, w5605) -> (w5609:errorcluster)
      }
      frame "Test Channel 9C" {
        w5653 = T9 {"command"="", "data"=variant} ("element")
        w5674 = T9 {"command"="", "data"=variant} ("element")
        w5695 = 9  # DUT channel (1-10)
        n2410 = disable-structure shown="LOGGING==TRUE" {
          disable-tunnel: w5690 -> [w5721 _]
          frame condition #0 (active) {
            n2411 = Empty String/Path?(string/path=w5721) -> (empty?=w5723:bool)
            n2412 = Select(t="Quece timeout", s=w5723, f=w5721) -> (s? t:f=w5720:string)
            n2413 = call "string log (SubVI).vi"("state Name"=w5720) -> ()  [unwired: 9 in, 2 out]
          }
          frame condition #1 {
          }
        }
        n2414 = Bundle By Name(cluster=w5674, "command"="Apps.UI Update", "data"="C") -> (w5673:T9)
        n2415 = Bundle By Name(cluster=w5674, "command"="MEAS.AllRelaysOFF2") -> (w5672:T9)
        n2416 = Bundle By Name(cluster=w5674, "command"="Apps.WaitForEvent") -> (w5671:T9)
        n2417 = Build Array(w5673, w5672, w5671) -> (w5679:T9[])
        n2418 = for {
          tunnel: [w5711] -> w5685 mode=indexing
          shift-right: [w5712] -> w5687
          shift-left: w5680 -> [w5710]
          tunnel: w5679 -> [w5709] mode=indexing
          n2419 = Unbundle By Name(w5709) -> ("command"=w5708:string, "data"=w5707:variant)
          n2420 = call "App enquece.vi"("Priority Enquece"=TRUE, "command data"=w5707, "command"=w5708, "queue in"=w5710) -> ("error out"=w5711:errorcluster, "Queue out"=w5712:refnum<queue>)  [unwired: 6 in]
        }
        n2421 = call "FGV DRV stand.vi"() -> ("Sub-Test.DCV"=w5668:bool)  [unwired: 10 in, 1 out]
        n2422 = case shown="True" w5668 {
          tunnel: [w5698 w5706] -> w5688
          frame False {
            n2423 = Build Array("WaitFor", "MEAS.requestAC") -> (w5698:string[])
          }
          frame True {
            n2424 = Build Array("Test DRV 49", "Test DRV 50", "Test DRV 51", "WaitForC", "MEAS.requestAC") -> (w5706:string[])
          }
        }
        n2425 = Merge Errors(w5685) -> (w5678:errorcluster)
        n2426 = Reverse 1D Array(array=w5688) -> (reversed array=w5667:string[])
        n2427 = for {
          tunnel: w5667 -> [w5718] mode=indexing
          tunnel: [w5717] -> w5684 mode=indexing
          shift-right: [w5716] -> w5686
          shift-left: w5687 -> [w5719]
          tunnel: w5678 -> [w5715]
          n2428 = call "App enquece.vi"("Priority Enquece"=TRUE, "error in (no error)"=w5715, "command"=w5718, "queue in"=w5719) -> ("error out"=w5717:errorcluster, "Queue out"=w5716:refnum<queue>)  [unwired: 6 in]
        }
        n2429 = Initialize Array(FALSE ("element"), 6 ("dimension size")) -> (w5649:bool[])
        n2430 = Merge Errors(w5684) -> (w5683:errorcluster)
        n2431 = Initialize Array(TRUE, 3 ("dimension size")) -> (w5648:bool[])
        n2432 = Replace Array Subset(array=w5649, new element=w5648) -> (w5647:bool[])  [unwired: 1 in]
        n2433 = To Variant(anything=T3."mux10_1_channel9" ("mux10_1(x6)_encode")) -> (Variant=w5664:variant)
        n2434 = To Variant(anything=T4."demux1_10_channel9" ("demux1_10(x6)_encode")) -> (Variant=w5660:variant)
        n2435 = To Variant(anything=w5647) -> (Variant=w5656:variant)
        n2436 = Bundle By Name(cluster=w5653, "command"="MEAS.mux10-1", "data"=w5664) -> (w5659:T9)
        n2437 = Bundle By Name(cluster=w5653, "command"="MEAS.demux1-10", "data"=w5660) -> (w5658:T9)
        n2438 = Bundle By Name(cluster=w5653, "command"="MEAS.eMIC", "data"=w5656) -> (w5655:T9)
        n2439 = Build Array(w5659, w5658, w5655) -> (w5682:T9[])
        n2440 = Reverse 1D Array(array=w5682) -> (reversed array=w5681:T9[])
        n2441 = for {
          tunnel: w5681 -> [w5729] mode=indexing
          tunnel: [w5726] -> w5689 mode=indexing
          tunnel: w5683 -> [w5725]
          tunnel: w5686 -> [w5730]
          n2442 = Unbundle By Name(w5729) -> ("command"=w5728:string, "data"=w5727:variant)
          n2443 = call "App enquece.vi"("Priority Enquece"=TRUE, "error in (no error)"=w5725, "command data"=w5727, "command"=w5728, "queue in"=w5730) -> ("error out"=w5726:errorcluster)  [unwired: 5 in, 1 out]
        }
        n2444 = Merge Errors(w5692, w5689) -> (w5693:errorcluster)
      }
      frame "Test Channel 10D" {
        w5737 = T9 {"command"="", "data"=variant} ("element")
        w5758 = T9 {"command"="", "data"=variant} ("element")
        w5779 = 10  # DUT channel (1-10)
        n2445 = disable-structure shown="LOGGING==TRUE" {
          disable-tunnel: w5774 -> [w5806 _]
          frame condition #0 (active) {
            n2446 = Empty String/Path?(string/path=w5806) -> (empty?=w5808:bool)
            n2447 = Select(t="Quece timeout", s=w5808, f=w5806) -> (s? t:f=w5805:string)
            n2448 = call "string log (SubVI).vi"("state Name"=w5805) -> ()  [unwired: 9 in, 2 out]
          }
          frame condition #1 {
          }
        }
        n2449 = Bundle By Name(cluster=w5758, "command"="Apps.UI Update", "data"="D") -> (w5757:T9)
        n2450 = Bundle By Name(cluster=w5758, "command"="MEAS.AllRelaysOFF2") -> (w5751:T9)
        n2451 = Bundle By Name(cluster=w5758, "command"="Apps.WaitForEvent") -> (w5756:T9)
        n2452 = Build Array(w5757, w5751, w5756) -> (w5763:T9[])
        n2453 = for {
          tunnel: [w5796] -> w5769 mode=indexing
          shift-right: [w5797] -> w5771
          shift-left: w5764 -> [w5795]
          tunnel: w5763 -> [w5794] mode=indexing
          n2454 = Unbundle By Name(w5794) -> ("command"=w5793:string, "data"=w5792:variant)
          n2455 = call "App enquece.vi"("Priority Enquece"=TRUE, "command data"=w5792, "command"=w5793, "queue in"=w5795) -> ("error out"=w5796:errorcluster, "Queue out"=w5797:refnum<queue>)  [unwired: 6 in]
        }
        n2456 = call "FGV DRV stand.vi"() -> ("Sub-Test.DCV"=w5752:bool)  [unwired: 10 in, 1 out]
        n2457 = case shown="True" w5752 {
          tunnel: [w5782 w5791] -> w5772
          frame False {
            n2458 = Build Array("WaitFor", "MEAS.requestAC") -> (w5782:string[])
          }
          frame True {
            n2459 = Build Array("Test DRV 55", "Test DRV 56", "Test DRV 57", "Test DRV 58", "WaitForD", "MEAS.requestAC") -> (w5791:string[])
          }
        }
        n2460 = Merge Errors(w5769) -> (w5762:errorcluster)
        n2461 = Reverse 1D Array(array=w5772) -> (reversed array=w5750:string[])
        n2462 = for {
          tunnel: w5750 -> [w5803] mode=indexing
          tunnel: [w5802] -> w5768 mode=indexing
          shift-right: [w5801] -> w5770
          shift-left: w5771 -> [w5804]
          tunnel: w5762 -> [w5800]
          n2463 = call "App enquece.vi"("Priority Enquece"=TRUE, "error in (no error)"=w5800, "command"=w5803, "queue in"=w5804) -> ("error out"=w5802:errorcluster, "Queue out"=w5801:refnum<queue>)  [unwired: 6 in]
        }
        n2464 = Initialize Array(FALSE ("element"), 6 ("dimension size")) -> (w5733:bool[])
        n2465 = Initialize Array(TRUE, 4 ("dimension size")) -> (w5732:bool[])
        n2466 = Merge Errors(w5768) -> (w5767:errorcluster)
        n2467 = Replace Array Subset(array=w5733, new element=w5732) -> (w5731:bool[])  [unwired: 1 in]
        n2468 = To Variant(anything=T3."mux10_1_channel10" ("mux10_1(x6)_encode")) -> (Variant=w5748:variant)
        n2469 = To Variant(anything=T4."demux1_10_channel10" ("demux1_10(x6)_encode")) -> (Variant=w5744:variant)
        n2470 = To Variant(anything=w5731) -> (Variant=w5740:variant)
        n2471 = Bundle By Name(cluster=w5737, "command"="MEAS.mux10-1", "data"=w5748) -> (w5743:T9)
        n2472 = Bundle By Name(cluster=w5737, "command"="MEAS.demux1-10", "data"=w5744) -> (w5742:T9)
        n2473 = Bundle By Name(cluster=w5737, "command"="MEAS.eMIC", "data"=w5740) -> (w5739:T9)
        n2474 = Build Array(w5743, w5742, w5739) -> (w5766:T9[])
        n2475 = Reverse 1D Array(array=w5766) -> (reversed array=w5765:T9[])
        n2476 = for {
          tunnel: w5765 -> [w5814] mode=indexing
          tunnel: [w5811] -> w5773 mode=indexing
          tunnel: w5767 -> [w5810]
          tunnel: w5770 -> [w5815]
          n2477 = Unbundle By Name(w5814) -> ("command"=w5813:string, "data"=w5812:variant)
          n2478 = call "App enquece.vi"("Priority Enquece"=TRUE, "error in (no error)"=w5810, "command data"=w5812, "command"=w5813, "queue in"=w5815) -> ("error out"=w5811:errorcluster)  [unwired: 5 in, 1 out]
        }
        n2479 = Merge Errors(w5776, w5773) -> (w5777:errorcluster)
      }
      frame "Test Channel 1D" {
        w5822 = T9 {"command"="", "data"=variant} ("element")
        w5843 = T9 {"command"="", "data"=variant} ("element")
        w5864 = 1  # DUT channel (1-10)
        n2480 = disable-structure shown="LOGGING==TRUE" {
          disable-tunnel: w5859 -> [w5891 _]
          frame condition #0 (active) {
            n2481 = Empty String/Path?(string/path=w5891) -> (empty?=w5893:bool)
            n2482 = Select(t="Quece timeout", s=w5893, f=w5891) -> (s? t:f=w5890:string)
            n2483 = call "string log (SubVI).vi"("state Name"=w5890) -> ()  [unwired: 9 in, 2 out]
          }
          frame condition #1 {
          }
        }
        n2484 = Bundle By Name(cluster=w5843, "command"="Apps.WaitForEvent") -> (w5841:T9)
        n2485 = Bundle By Name(cluster=w5843, "command"="Apps.UI Update", "data"="D") -> (w5842:T9)
        n2486 = Bundle By Name(cluster=w5843, "command"="MEAS.AllRelaysOFF2") -> (w5836:T9)
        n2487 = Build Array(w5842, w5836, w5841) -> (w5848:T9[])
        n2488 = for {
          tunnel: [w5881] -> w5854 mode=indexing
          shift-right: [w5882] -> w5856
          shift-left: w5849 -> [w5880]
          tunnel: w5848 -> [w5879] mode=indexing
          n2489 = Unbundle By Name(w5879) -> ("command"=w5878:string, "data"=w5877:variant)
          n2490 = call "App enquece.vi"("Priority Enquece"=TRUE, "command data"=w5877, "command"=w5878, "queue in"=w5880) -> ("error out"=w5881:errorcluster, "Queue out"=w5882:refnum<queue>)  [unwired: 6 in]
        }
        n2491 = call "FGV DRV stand.vi"() -> ("Sub-Test.DCV"=w5837:bool)  [unwired: 10 in, 1 out]
        n2492 = case shown="True" w5837 {
          tunnel: [w5867 w5876] -> w5857
          frame False {
            n2493 = Build Array("WaitFor", "MEAS.requestAC") -> (w5867:string[])
          }
          frame True {
            n2494 = Build Array("Test DRV 1", "Test DRV 2", "Test DRV 3", "Test DRV 4", "WaitForD", "MEAS.requestAC") -> (w5876:string[])
          }
        }
        n2495 = Merge Errors(w5854) -> (w5847:errorcluster)
        n2496 = Reverse 1D Array(array=w5857) -> (reversed array=w5835:string[])
        n2497 = for {
          tunnel: w5835 -> [w5888] mode=indexing
          tunnel: [w5887] -> w5853 mode=indexing
          shift-right: [w5886] -> w5855
          shift-left: w5856 -> [w5889]
          tunnel: w5847 -> [w5885]
          n2498 = call "App enquece.vi"("Priority Enquece"=TRUE, "error in (no error)"=w5885, "command"=w5888, "queue in"=w5889) -> ("error out"=w5887:errorcluster, "Queue out"=w5886:refnum<queue>)  [unwired: 6 in]
        }
        n2499 = Merge Errors(w5853) -> (w5852:errorcluster)
        n2500 = Initialize Array(FALSE ("element"), 6 ("dimension size")) -> (w5818:bool[])
        n2501 = Initialize Array(TRUE, 4 ("dimension size")) -> (w5817:bool[])
        n2502 = Replace Array Subset(array=w5818, new element=w5817) -> (w5816:bool[])  [unwired: 1 in]
        n2503 = To Variant(anything=T3."mux10_1_channel1" ("mux10_1(x6)_encode")) -> (Variant=w5833:variant)
        n2504 = To Variant(anything=T4."demux1_10_channel1" ("demux1_10(x6)_encode")) -> (Variant=w5829:variant)
        n2505 = To Variant(anything=w5816) -> (Variant=w5825:variant)
        n2506 = Bundle By Name(cluster=w5822, "command"="MEAS.mux10-1", "data"=w5833) -> (w5828:T9)
        n2507 = Bundle By Name(cluster=w5822, "command"="MEAS.demux1-10", "data"=w5829) -> (w5827:T9)
        n2508 = Bundle By Name(cluster=w5822, "command"="MEAS.eMIC", "data"=w5825) -> (w5824:T9)
        n2509 = Build Array(w5828, w5827, w5824) -> (w5851:T9[])
        n2510 = Reverse 1D Array(array=w5851) -> (reversed array=w5850:T9[])
        n2511 = for {
          tunnel: w5850 -> [w5899] mode=indexing
          tunnel: [w5896] -> w5858 mode=indexing
          tunnel: w5852 -> [w5895]
          tunnel: w5855 -> [w5900]
          n2512 = Unbundle By Name(w5899) -> ("command"=w5898:string, "data"=w5897:variant)
          n2513 = call "App enquece.vi"("Priority Enquece"=TRUE, "error in (no error)"=w5895, "command data"=w5897, "command"=w5898, "queue in"=w5900) -> ("error out"=w5896:errorcluster)  [unwired: 5 in, 1 out]
        }
        n2514 = Merge Errors(w5861, w5858) -> (w5862:errorcluster)
      }
      frame "Test Channel 2D" {
        w5907 = T9 {"command"="", "data"=variant} ("element")
        w5928 = T9 {"command"="", "data"=variant} ("element")
        w5949 = 2  # DUT channel (1-10)
        n2515 = disable-structure shown="LOGGING==TRUE" {
          disable-tunnel: w5944 -> [w5976 _]
          frame condition #0 (active) {
            n2516 = Empty String/Path?(string/path=w5976) -> (empty?=w5978:bool)
            n2517 = Select(t="Quece timeout", s=w5978, f=w5976) -> (s? t:f=w5975:string)
            n2518 = call "string log (SubVI).vi"("state Name"=w5975) -> ()  [unwired: 9 in, 2 out]
          }
          frame condition #1 {
          }
        }
        n2519 = Bundle By Name(cluster=w5928, "command"="Apps.WaitForEvent") -> (w5926:T9)
        n2520 = Bundle By Name(cluster=w5928, "command"="Apps.UI Update", "data"="D") -> (w5927:T9)
        n2521 = Bundle By Name(cluster=w5928, "command"="MEAS.AllRelaysOFF2") -> (w5921:T9)
        n2522 = Build Array(w5927, w5921, w5926) -> (w5933:T9[])
        n2523 = for {
          tunnel: [w5966] -> w5939 mode=indexing
          shift-right: [w5967] -> w5941
          shift-left: w5934 -> [w5965]
          tunnel: w5933 -> [w5964] mode=indexing
          n2524 = Unbundle By Name(w5964) -> ("command"=w5963:string, "data"=w5962:variant)
          n2525 = call "App enquece.vi"("Priority Enquece"=TRUE, "command data"=w5962, "command"=w5963, "queue in"=w5965) -> ("error out"=w5966:errorcluster, "Queue out"=w5967:refnum<queue>)  [unwired: 6 in]
        }
        n2526 = call "FGV DRV stand.vi"() -> ("Sub-Test.DCV"=w5922:bool)  [unwired: 10 in, 1 out]
        n2527 = case shown="True" w5922 {
          tunnel: [w5952 w5961] -> w5942
          frame False {
            n2528 = Build Array("WaitFor", "MEAS.requestAC") -> (w5952:string[])
          }
          frame True {
            n2529 = Build Array("Test DRV 7", "Test DRV 8", "Test DRV 9", "Test DRV 10", "WaitForD", "MEAS.requestAC") -> (w5961:string[])
          }
        }
        n2530 = Merge Errors(w5939) -> (w5932:errorcluster)
        n2531 = Reverse 1D Array(array=w5942) -> (reversed array=w5920:string[])
        n2532 = for {
          tunnel: w5920 -> [w5973] mode=indexing
          tunnel: [w5972] -> w5938 mode=indexing
          shift-right: [w5971] -> w5940
          shift-left: w5941 -> [w5974]
          tunnel: w5932 -> [w5970]
          n2533 = call "App enquece.vi"("Priority Enquece"=TRUE, "error in (no error)"=w5970, "command"=w5973, "queue in"=w5974) -> ("error out"=w5972:errorcluster, "Queue out"=w5971:refnum<queue>)  [unwired: 6 in]
        }
        n2534 = Initialize Array(FALSE ("element"), 6 ("dimension size")) -> (w5903:bool[])
        n2535 = Initialize Array(TRUE, 4 ("dimension size")) -> (w5902:bool[])
        n2536 = Merge Errors(w5938) -> (w5937:errorcluster)
        n2537 = Replace Array Subset(array=w5903, new element=w5902) -> (w5901:bool[])  [unwired: 1 in]
        n2538 = To Variant(anything=T3."mux10_1_channel2" ("mux10_1(x6)_encode")) -> (Variant=w5918:variant)
        n2539 = To Variant(anything=T4."demux1_10_channel2" ("demux1_10(x6)_encode")) -> (Variant=w5914:variant)
        n2540 = To Variant(anything=w5901) -> (Variant=w5910:variant)
        n2541 = Bundle By Name(cluster=w5907, "command"="MEAS.mux10-1", "data"=w5918) -> (w5913:T9)
        n2542 = Bundle By Name(cluster=w5907, "command"="MEAS.demux1-10", "data"=w5914) -> (w5912:T9)
        n2543 = Bundle By Name(cluster=w5907, "command"="MEAS.eMIC", "data"=w5910) -> (w5909:T9)
        n2544 = Build Array(w5913, w5912, w5909) -> (w5936:T9[])
        n2545 = Reverse 1D Array(array=w5936) -> (reversed array=w5935:T9[])
        n2546 = for {
          tunnel: w5935 -> [w5984] mode=indexing
          tunnel: [w5981] -> w5943 mode=indexing
          tunnel: w5937 -> [w5980]
          tunnel: w5940 -> [w5985]
          n2547 = Unbundle By Name(w5984) -> ("command"=w5983:string, "data"=w5982:variant)
          n2548 = call "App enquece.vi"("Priority Enquece"=TRUE, "error in (no error)"=w5980, "command data"=w5982, "command"=w5983, "queue in"=w5985) -> ("error out"=w5981:errorcluster)  [unwired: 5 in, 1 out]
        }
        n2549 = Merge Errors(w5946, w5943) -> (w5947:errorcluster)
      }
      frame "Test Channel 3D" {
        w5992 = T9 {"command"="", "data"=variant} ("element")
        w6013 = T9 {"command"="", "data"=variant} ("element")
        w6034 = 3  # DUT channel (1-10)
        n2550 = disable-structure shown="LOGGING==TRUE" {
          disable-tunnel: w6029 -> [w6061 _]
          frame condition #0 (active) {
            n2551 = Empty String/Path?(string/path=w6061) -> (empty?=w6063:bool)
            n2552 = Select(t="Quece timeout", s=w6063, f=w6061) -> (s? t:f=w6060:string)
            n2553 = call "string log (SubVI).vi"("state Name"=w6060) -> ()  [unwired: 9 in, 2 out]
          }
          frame condition #1 {
          }
        }
        n2554 = Bundle By Name(cluster=w6013, "command"="Apps.WaitForEvent") -> (w6011:T9)
        n2555 = Bundle By Name(cluster=w6013, "command"="Apps.UI Update", "data"="D") -> (w6012:T9)
        n2556 = Bundle By Name(cluster=w6013, "command"="MEAS.AllRelaysOFF2") -> (w6006:T9)
        n2557 = Build Array(w6012, w6006, w6011) -> (w6018:T9[])
        n2558 = for {
          tunnel: [w6051] -> w6024 mode=indexing
          shift-right: [w6052] -> w6026
          shift-left: w6019 -> [w6050]
          tunnel: w6018 -> [w6049] mode=indexing
          n2559 = Unbundle By Name(w6049) -> ("command"=w6048:string, "data"=w6047:variant)
          n2560 = call "App enquece.vi"("Priority Enquece"=TRUE, "command data"=w6047, "command"=w6048, "queue in"=w6050) -> ("error out"=w6051:errorcluster, "Queue out"=w6052:refnum<queue>)  [unwired: 6 in]
        }
        n2561 = call "FGV DRV stand.vi"() -> ("Sub-Test.DCV"=w6007:bool)  [unwired: 10 in, 1 out]
        n2562 = case shown="True" w6007 {
          tunnel: [w6037 w6046] -> w6027
          frame False {
            n2563 = Build Array("WaitFor", "MEAS.requestAC") -> (w6037:string[])
          }
          frame True {
            n2564 = Build Array("Test DRV 13", "Test DRV 14", "Test DRV 15", "Test DRV 16", "WaitForD", "MEAS.requestAC") -> (w6046:string[])
          }
        }
        n2565 = Merge Errors(w6024) -> (w6017:errorcluster)
        n2566 = Reverse 1D Array(array=w6027) -> (reversed array=w6005:string[])
        n2567 = for {
          tunnel: w6005 -> [w6058] mode=indexing
          tunnel: [w6057] -> w6023 mode=indexing
          shift-right: [w6056] -> w6025
          shift-left: w6026 -> [w6059]
          tunnel: w6017 -> [w6055]
          n2568 = call "App enquece.vi"("Priority Enquece"=TRUE, "error in (no error)"=w6055, "command"=w6058, "queue in"=w6059) -> ("error out"=w6057:errorcluster, "Queue out"=w6056:refnum<queue>)  [unwired: 6 in]
        }
        n2569 = Initialize Array(FALSE ("element"), 6 ("dimension size")) -> (w5988:bool[])
        n2570 = Initialize Array(TRUE, 4 ("dimension size")) -> (w5987:bool[])
        n2571 = Merge Errors(w6023) -> (w6022:errorcluster)
